vi "task7_CASE_STRUCTURE.vi"() -> ()   [LabVIEW 2017]
panel:
  in  "Radio Buttons":enum32{"Octal", "Hexa", "Decimal", "Binary"}(radio)
  out "?":bool
  out "?":bool
  out "?":bool
  out "?":bool
  out "?":bool
  out "?":bool
  out "?":bool
  out "?":bool
  in  "?":bool
  in  "?":bool
  in  "?":bool
  in  "?":bool
  in  "?":bool
  in  "?":bool
  in  "?":bool
  in  "?":bool
  out "output":string
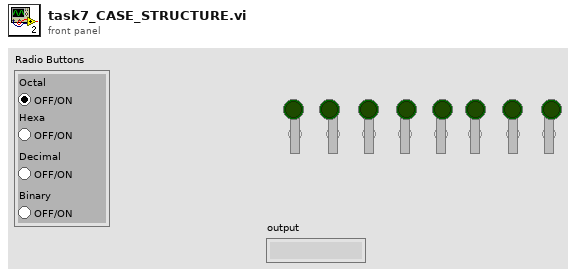
[diagram p1: front panel]
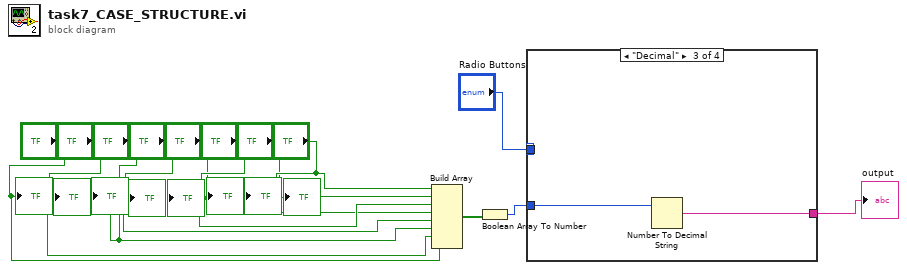
[diagram p0: block diagram]
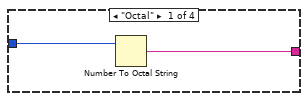
[diagram p2: hidden frame]
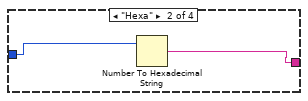
[diagram p3: hidden frame]
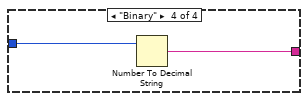
[diagram p4: hidden frame]
diagram:
  n1 = Build Array("?", "?", "?", "?", "?", "?", "?", "?") -> (w4:bool[])
  n2 = Boolean Array To Number(Boolean array=w4) -> (number=w3:u32)
  n3 = case shown="\"Decimal\"" "Radio Buttons" {
    selector: "Radio Buttons" -> [_ _ w19 _]
    tunnel: [_ _ w19 _] -> _
    tunnel: w3 -> [w14 w16 w18 w21]
    tunnel: [w13 w15 w17 w20] -> w1
    frame "Octal" {
      n4 = Number To Octal String(2:w14) -> (0:w13:string)  [unwired: 1 in]
    }
    frame "Hexa" {
      n5 = Number To Hexadecimal String(2:w16) -> (0:w15:string)  [unwired: 1 in]
    }
    frame "Decimal" {
      n6 = Number To Decimal String(number=w18) -> (decimal integer string=w17:string)  [unwired: 1 in]
    }
    frame "Binary" {
      n7 = Number To Decimal String(number=w21) -> (decimal integer string=w20:string)  [unwired: 1 in]
    }
  }
  "output" <- w1
  "?" <- "?"
  "?" <- "?"
  "?" <- "?"
  "?" <- "?"
  "?" <- "?"
  "?" <- "?"
  "?" <- "?"
  "?" <- "?"
